vi "LogVICall(Caller).vi"(8 "Error In":errorcluster, 11 "Caller VI":refnum<vi>) -> (0 "Error Out":errorcluster)   [LabVIEW 2019, in "EventLogger.lvlib"]
uses:
  EventLogger.lvlib
  Enum - Message.ctl
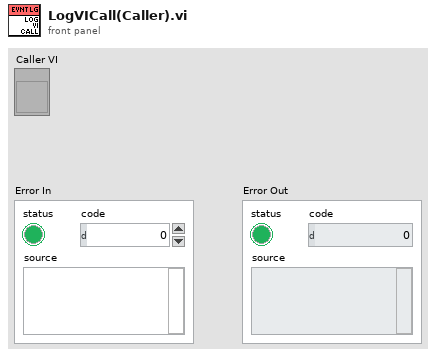
[diagram p1: front panel]
types:
  T1 = typedef "EventLogger.lvlib/Enum - Message.ctl" = enum16{"Initialize", "Idle", "CreateLog", "LogStrEvent", "LogErrorEvent", "LogVICall", "Error", "Exit"}
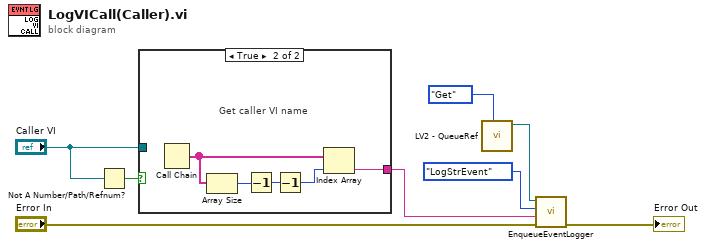
[diagram p0: block diagram]
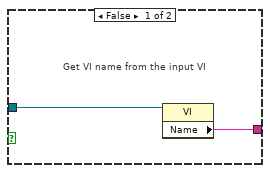
[diagram p2: hidden frame]
diagram:
  n1 = Not A Number/Path/Refnum?(number/path/refnum="Caller VI") -> (NaN/Path/Refnum?=w3:bool)
  n2 = case shown="True" w3 {
    tunnel: "Caller VI" -> [w10 _]
    tunnel: [w9 w12] -> w1
    frame False {
      # "Get VI name from the input VI"
      n3 = property class="VI"(reference=w10) -> ("Name"=w9:string)  [unwired: 1 in, 2 out]
    }
    frame True {
      # "Get caller VI name"
      n4 = Call Chain() -> (call chain=w14:string[])
      n5 = Array Size(array=w14) -> (size(s)=w13:i32)
      n6 = Decrement(x=w13) -> (x-1=w15:i32)
      n7 = Decrement(x=w15) -> (x-1=w11:i32)
      n8 = Index Array(array=w14, index=w11) -> (element=w12:string)
    }
  }
  n9 = call "LV2 - QueueRef.vi"("Action"=enum16{"Set", "Get"}."Get") -> ("EventLoggerQueue out"=w6:refnum<queue>)  [unwired: 10 in]
  n10 = call "EnqueueEventLogger.vi"("Error In"="Error In", "Data"=w1, "Message"=Enum_-_Message."LogStrEvent", "EventLoggerQueue"=w6) -> ("Error Out"=→"Error Out":errorcluster)  [unwired: 6 in, 1 out]
